vi "mask.vi"(8 "error in (no error)":errorcluster, 9 "mask channel":u8=253 format="%b", 10 "Address":u32, 11 "IP address":string="192.168.10.21") -> (0 "error out":errorcluster)   [LabVIEW 2017]
panel:
  in  "Read (TRUE)":bool
  out "Out":u8=253 format="%.0x"
  in  "MASK_1":bool=TRUE
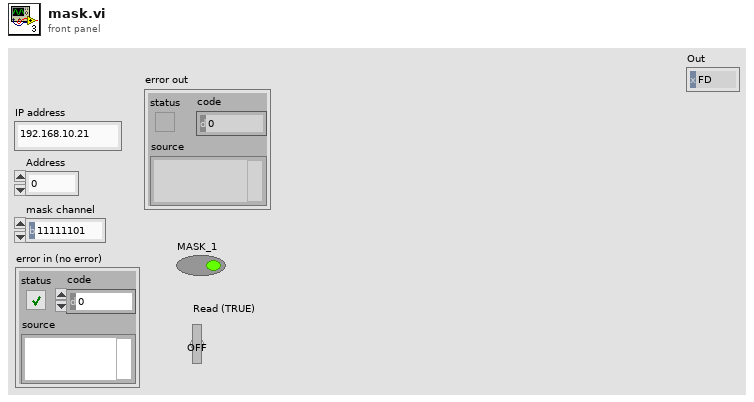
[diagram p1: front panel]
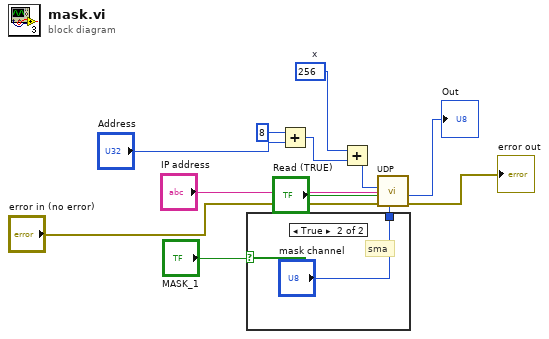
[diagram p0: block diagram]
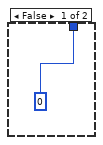
[diagram p2: hidden frame]
diagram:
  w10 = u16 256  # x
  n1 = case shown="True" "MASK_1" {
    tunnel: [u8 0 ("In") "mask channel"] -> w12
    frame False {
    }
    frame True {
      # "sma"
    }
  }
  n2 = Add(x=u8 8, y="Address") -> (x+y=w4:u32)
  n3 = Add(x=w10, y=w4) -> (x+y=w9:u32)
  n4 = call "UDP.vi"("In"=w12, "error in (no error)"="error in (no error)", "Read (TRUE)"="Read (TRUE)", "Address"=w9, "IP address"="IP address") -> ("error out"=→"error out":errorcluster, "Out"=→"Out":u8)  [unwired: 3 in, 1 out]
